vi "Write CAN FIFO Direct Dispatch.vi"(6 "FIFO Timestamps":T1, 8 "error in (no error)":errorcluster, 9 "Timeout (ms)":i32, 10 "Data":u8[](array[numeric]) format="%.0x", 11 "CIFTag in":refnum<class "CIFChannels.lvclass">) -> (0 "error out":errorcluster, 1 "timed out?":bool, 3 "CIFTag out":refnum<class "CIF_NIChn_FifoCAN.lvclass">)   [LabVIEW 2021, in "CIF_NIChn_FifoCAN.lvclass"]
uses:
  CIF_NIChn_FifoCAN.lvclass
  CIF_NIChn_FifoCAN.lvclass/CIF_NIChn_FifoCAN.ctl
  NIChn/CIF_NIChn.lvclass
  <vilib>/CIF Foundation/CIF Channels/CIFChannels/CIFChannelCore.lvlib
  ChannelCommon/CIFFIFO/CIFfifo.lvclass
  D:/dev/Packages/Channel_Manager/src/CIF_NIChn/NIChn/CIF_NIChn.lvclass
  D:/dev/Packages/Channel_Manager/src/CIFChannels/CIFChannels.lvclass
  D:/dev/Packages/Channel_Manager/src/CIF_NIChn/FIFO_CAN/CIF_NIChn_FifoCAN.lvclass
  CIFChannels/CIFChannels.lvclass
  ChannelCommon/typedef/TimeStamps.ctl
  ChannelCommon/ChannelCommon.lvlib
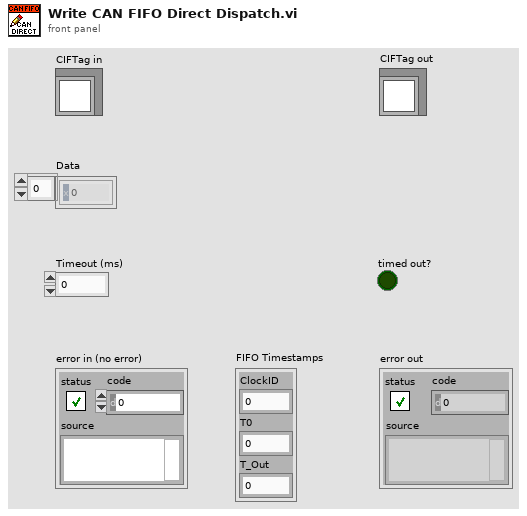
[diagram p1: front panel]
types:
  T1 = typedef "ChannelCommon.lvlib/TimeStamps.ctl" = cluster{"ClockID":u8, "T0":i64, "T_Out":i64}
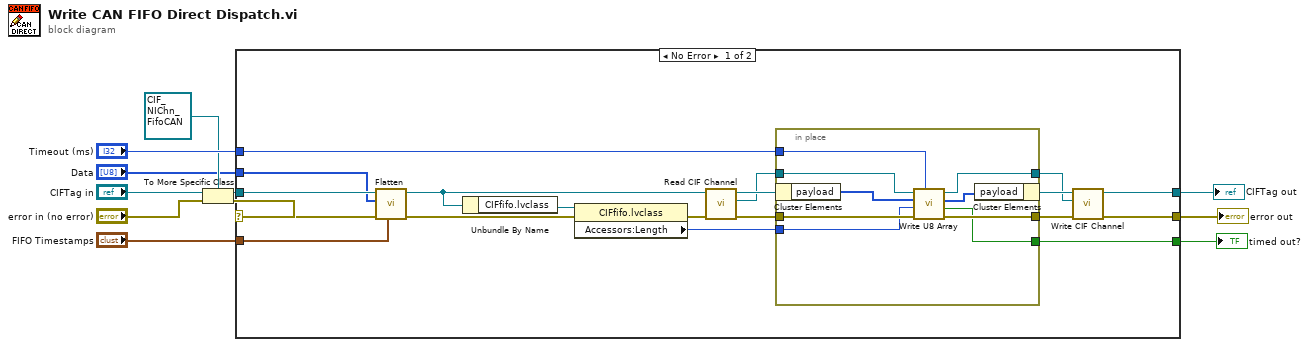
[diagram p0: block diagram]
diagram:
  n1 = To More Specific Class(target class=refnum<class "CIF_NIChn_FifoCAN.lvclass"> refnum ("CIFTag in"), reference="CIFTag in", error in="error in (no error)") -> (specific class reference=w5:refnum<class "CIF_NIChn_FifoCAN.lvclass">, error out=w3:errorcluster)
  n2 = case shown="No Error" w3 {
    selector: w3 -> [w14 w41]
    tunnel: [w21 w41] -> w11
    tunnel: [w26 w40] -> w10
    tunnel: w5 -> [w18 w40]
    tunnel: [w30 _] -> w9
    tunnel: "Timeout (ms)" -> [w22 _]
    tunnel: "Data" -> [w15 _]
    tunnel: "FIFO Timestamps" -> [w12 _]
    frame No Error {
      n3 = call "Flatten.vi"("FIFO Timestamps"=w12, "error in (no error)"=w14, "Data in"=w15, "CIFTag in"=w18) -> ("error out"=w16:errorcluster, "CIFTag out"=w17:refnum<class "CIF_NIChn_FifoCAN.lvclass">)  [unwired: 6 in]
      n4 = Unbundle By Name(w17) -> ("CIFfifo.lvclass"=w20:refnum<class "CIFfifo.lvclass">)
      n5 = property class="CIFfifo.lvclass"(reference=w20, error in=w16) -> (error out=w19:errorcluster, "Accessors:Length"=w13:u64)  [unwired: 1 out]
      n6 = call "Read CIF Channel.vi"("error in (no error)"=w19, "CIFTag in"=w17) -> ("error out"=w28:errorcluster, "CIF Channel"=w24:refnum<k21>, "CIFTag out"=w29:refnum<class "CIF_NIChn_FifoCAN.lvclass">)  [unwired: 7 in]
      n7 = in-place {
        in-place-border: w28 -> [w39]
        in-place-border: [w38] -> w25
        in-place-border: [w37] -> w30
        in-place-border: w24 -> [w36]
        in-place-border: [w35] -> w23
        in-place-border: w22 -> [w34]
        in-place-border: w13 -> [w32]
        n8 = in-place-cluster #1(w29) -> ("payload"=w33:u8[])
        n9 = call <vilib>:"Write U8 Array.vi"("Timeout (ms)"=w34, "error in"=w39, "Number of Elements"=w32, "U8 Array in"=w33, "CIF Channel in"=w36) -> ("error out"=w38:errorcluster, "Timed out?"=w37:bool, "U8 Array out"=w31:u8[], "CIF Channel out"=w35:refnum<k21>)  [unwired: 3 in]
        n10 = in-place-cluster #1("payload"=w31) -> (w27:refnum<class "CIF_NIChn_FifoCAN.lvclass">)
      }
      n11 = call "Write CIF Channel.vi"("error in (no error)"=w25, "CIF Channel"=w23, "CIFTag in"=w27) -> ("error out"=w21:errorcluster, "CIFTag out"=w26:refnum<class "CIF_NIChn_FifoCAN.lvclass">)  [unwired: 7 in]
    }
    frame Error {
    }
  }
  "error out" <- w11
  "CIFTag out" <- w10
  "timed out?" <- w9
